vi "Launch Object by Type Response.vi"(5 "Enqueuer":refnum<class "Message Enqueuer.lvclass">, 6 "Requestor":string, 8 "error in (no error)":errorcluster, 9 "Name":string, 10 "Type":string, 11 "Sequence Controller in":refnum<class "Sequence Controller.lvclass">) -> (0 "error out":errorcluster, 3 "Sequence Controller out":refnum<class "Sequence Controller.lvclass">)   [LabVIEW 2016, in "Sequence Controller.lvclass"]
uses:
  Sequence Controller.lvclass
  <vilib>/ActorFramework/Message Enqueuer/Message Enqueuer.lvclass
  Process Controller/Process Controller.lvclass
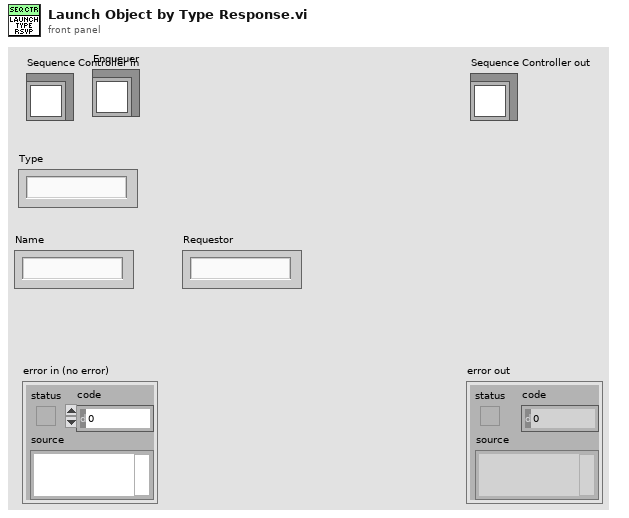
[diagram p1: front panel]
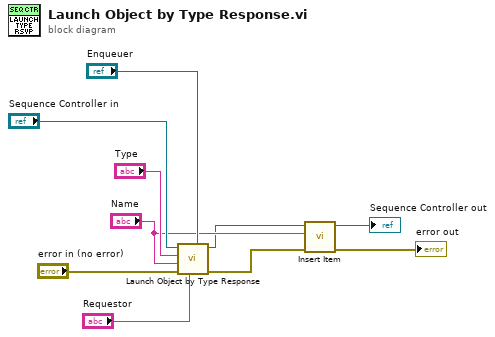
[diagram p0: block diagram]
diagram:
  n1 = call-parent "Launch Object by Type Response.vi"("Enqueuer"="Enqueuer", "Requestor"="Requestor", "error in (no error)"="error in (no error)", "Name"="Name", "Type"="Type", "Da Base in"="Sequence Controller in") -> ("error out"=w4:errorcluster, "Da Base out"=w2:refnum<class "Sequence Controller.lvclass">)  [unwired: 4 in]
  n2 = call-dynamic "Insert Item.vi"("error in (no error)"=w4, "Item"="Name", "Interactive Tree in"=w2) -> ("error out"=→"error out":errorcluster, "Interactive Tree out"=→"Sequence Controller out":refnum<class "Sequence Controller.lvclass">)  [unwired: 7 in]
